vi "3D Cartesian Coordinate Shift.vi"   [LabVIEW 2012, in "NI_AALPro.lvlib"]
doc: "Shifts three-dimensional Cartesian coordinates along the x-, y-, and z-axes. \n\nWire data to the <B>X</B> input to determine the polymorphic instance to use or manually select the instance."
uses:
  NI_AALPro.lvlib
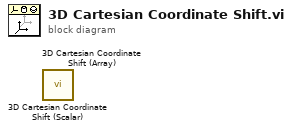
[diagram p0: block diagram]
diagram:
  n1 = call "3D Cartesian Coordinate Shift (Scalar).vi"() -> ()  [unwired: 8 in, 4 out]
  n2 = call "3D Cartesian Coordinate Shift (Array).vi"() -> ()  [unwired: 8 in, 4 out]
